vi "ke37xx Delete TSP Script.vi"(8 "error in (no error)":errorcluster, 10 "TSP Script Name to Delete":string, 11 "VISA Resource Name":refnum<visa-resource-name>) -> (0 "error out":errorcluster, 3 "VISA Resource Name Out":refnum<visa-resource-name>)   [LabVIEW 2009, in "Keithley 3700 Series.lvlib"]
doc: "This VI deletes a TSP Script stored on the instrument."
uses:
  <instrlib>/Keithley 3706/Keithley 3700 Series.lvlib
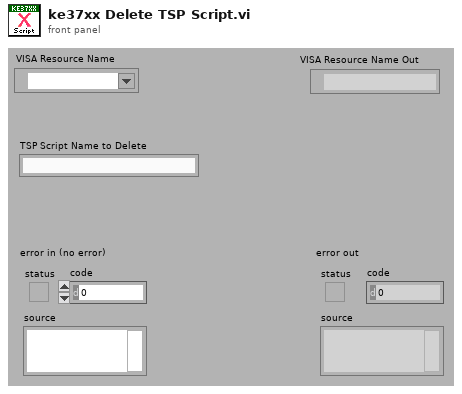
[diagram p1: front panel]
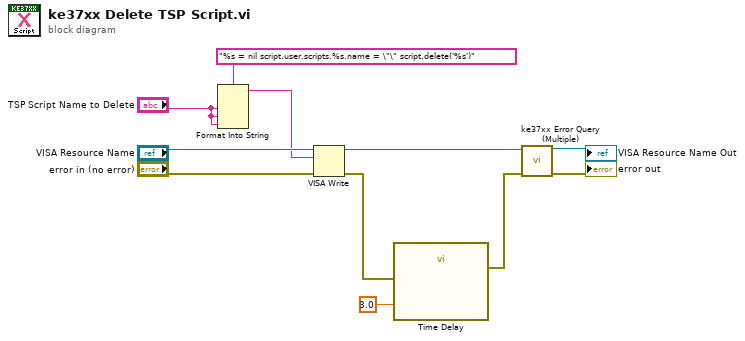
[diagram p0: block diagram]
diagram:
  n1 = Format Into String(format string="%s = nil script.user.scripts.%s.name = \"\" script.delete('%s')", "TSP Script Name to Delete", "TSP Script Name to Delete", "TSP Script Name to Delete") -> (resulting string=w5:string)  [unwired: 2 in, 1 out]
  n2 = VISA Write(VISA resource name="VISA Resource Name", write buffer=w5, error in (no error)="error in (no error)") -> (VISA resource name out=w7:refnum<visa-resource-name>, error out=w3:errorcluster)  [unwired: 1 out]
  n3 = call "Time Delay"("error in (no error)"=w3, "Delay Time (s)"=3.0) -> ("error out"=w2:errorcluster)  [unwired: 9 in]
  n4 = call <instrlib>:"ke37xx Error Query (Multiple).vi"("VISA resource name"=w7, "error in (no error)"=w2) -> ("VISA resource name out"=→"VISA Resource Name Out":refnum<visa-resource-name>, "error out"=→"error out":errorcluster)  [unwired: 12 out]
